vi "Set value by Variant.vi"(8 "error in (no error)":errorcluster, 10 "Variant":variant, 11 "Timestamp Column in":refnum<class "Timestamp Column.lvclass">) -> (0 "error out":errorcluster, 3 "Timestamp Column out":refnum<class "Timestamp Column.lvclass">)   [LabVIEW 2020, in "Basic Columns.lvlib" / "Timestamp Column.lvclass"]
uses:
  Timestamp Column.lvclass
  Timestamp Column.lvclass/Timestamp Column.ctl
  Column Interface/Timestamp Rule Interface/Timestamp Rule Interface.lvclass
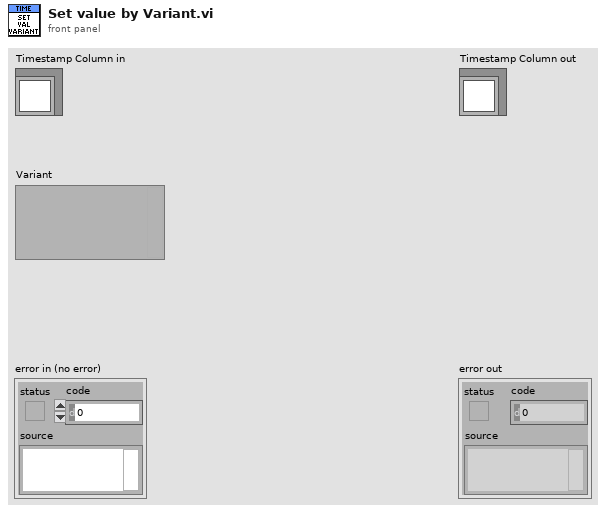
[diagram p1: front panel]
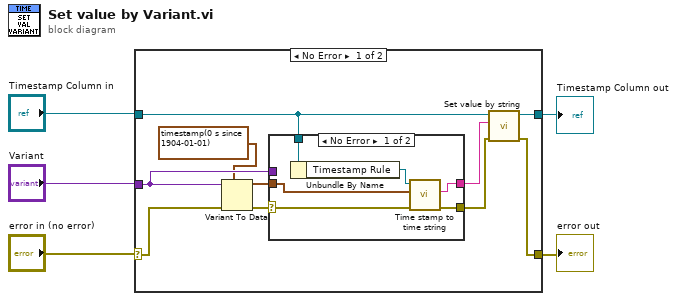
[diagram p0: block diagram]
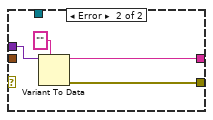
[diagram p2: hidden frame]
diagram:
  n1 = case shown="No Error" "error in (no error)" {
    selector: "error in (no error)" -> [w10 w27]
    tunnel: [w8 w27] -> w2
    tunnel: "Timestamp Column in" -> [w6 w26]
    tunnel: [w15 w26] -> w4
    tunnel: "Variant" -> [w12 _]
    frame No Error {
      n2 = Variant To Data(error in=w10, type=timestamp(0 s since 1904-01-01) ("Time Stamp"), Variant=w12) -> (data=w13:timestamp, error out=w14:errorcluster)
      n3 = case shown="No Error" w14 {
        selector: w14 -> [w20 _]
        tunnel: w13 -> [w17 _]
        tunnel: w12 -> [_ w25]
        tunnel: [w16 w23] -> w11
        tunnel: [w19 w22] -> w9
        tunnel: w6 -> [w21 _]
        frame No Error {
          n4 = Unbundle By Name(w21) -> ("Timestamp Rule"=w18:refnum<class "Timestamp Rule Interface.lvclass">)
          n5 = call-dynamic "Time stamp to time string.vi"("error in (no error)"=w20, "Time Stamp"=w17, "Timestamp Rule Interface in"=w18) -> ("error out"=w19:errorcluster, "String"=w16:string)  [unwired: 6 in, 1 out]
        }
        frame Error {
          n6 = Variant To Data(type="", Variant=w25) -> (data=w23:string, error out=w22:errorcluster)  [unwired: 1 in]
        }
      }
      n7 = call-dynamic "Set value by string.vi"("error in (no error)"=w9, "Value"=w11, "Column in"=w6) -> ("error out"=w8:errorcluster, "Column out"=w15:refnum<class "Timestamp Column.lvclass">)  [unwired: 7 in]
    }
    frame Error {
    }
  }
  "error out" <- w2
  "Timestamp Column out" <- w4
